vi "IPv4LL Numeric Address Constant.vi"() -> (3 "IPv4LL Subnet Address":u32)   [LabVIEW 2020, in "NI_WFCN.lvlib" / "IPv4 Network Address.lvclass"]
doc: "Returns IPv4LL subnet address (169.254.0.0) in native-byte-order U32 format."
uses:
  <vilib>/net/WFCN/Addressing/IPv4 Network Address/IPv4 Network Address.lvclass
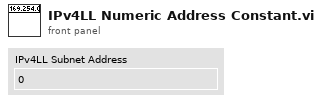
[diagram p1: front panel]
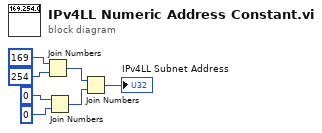
[diagram p0: block diagram]
diagram:
  n1 = Join Numbers(hi=u8 169 ("Numeric"), lo=u8 254 ("Numeric")) -> ((hi.lo)=w3:u16)
  n2 = Join Numbers(hi=u8 0 ("Numeric"), lo=u8 0 ("Numeric")) -> ((hi.lo)=w2:u16)
  n3 = Join Numbers(hi=w3, lo=w2) -> ((hi.lo)=→"IPv4LL Subnet Address":u32)
